vi "StringToPointer.vi"(3 "string":string) -> (0 "pointer":i32 format="%.0x")   [LabVIEW 2011]
doc: "Returns the pointer of the string. Compare with PointerToString.vi \nHex 00 in string is not passed.\n\nW.K. Walstra, © AIR Technical Automation bv\nwww.air.nl / info@air.nl (general info) / wiebe@air.nl (specific info)"
uses:
  KERNEL32.DLL
panel:
  # "nnnnn   nnn nnnnnn  \nnnnnnnn nnn nnnnnnn\nnnnnnnn nnn nnnnnnn\nnnnqnnn nnn nnn  nnn\nnnn  nnn nnn nnnnnnn\nnnn  nnn nnn nnnnnn  \nnnnnnnn nnn nnnnnnn\nnnnnnnn nnn nnn  nnn\nnnnnnnn nnn nnn  nnn\nnnn  nnn nnn nnn  nnn\nnnn  nnn nnn nnn  nnn"
  # "Technical Automation"
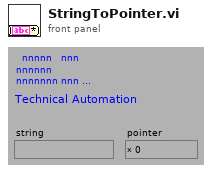
[diagram p1: front panel]
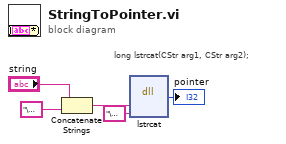
[diagram p0: block diagram]
diagram:
  # "long lstrcat(CStr arg1, CStr arg2);"
  n1 = Concatenate Strings("string", "\u0000") -> (w2:string)
  n2 = dll-call lib="KERNEL32.DLL" fn="lstrcat"(w2, "\u0000") -> (→"pointer":i32)  [unwired: 4 in, 3 out]
